vi "Scan for incomplete relaxations and re-submit script.vi"() -> ()   [LabVIEW 2010]
panel:
  in  "Move to other folder in source":bool
  in  "Target Directory":path=path "D:/Ab-initio/VASP Calcs/2D_Grain Boundaries/Batch25_20130914"
  in  "Source Directory":path=path "D:/Ab-initio/VASP Calcs/2D_Grain Boundaries/Batch18_20130828/A3B12_Periodic_Twin/CONTCAR"
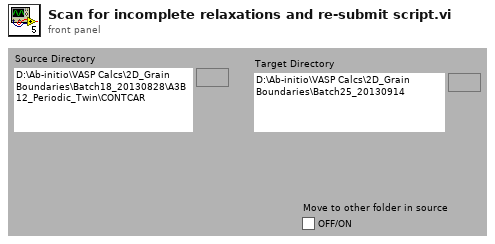
[diagram p1: front panel]
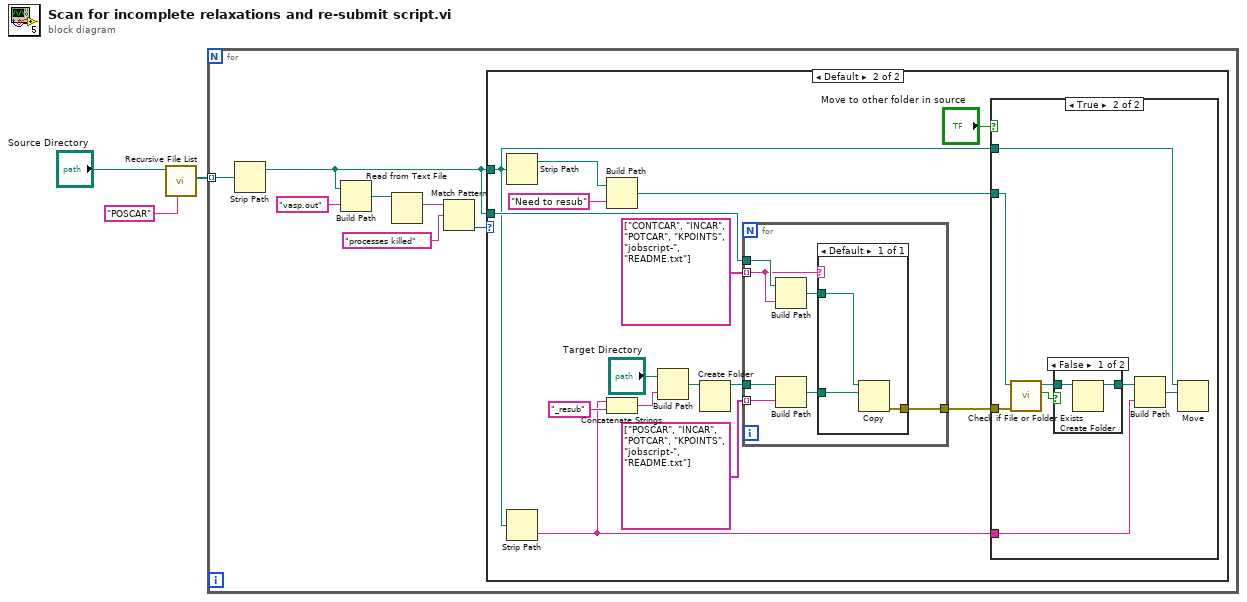
[diagram p0: block diagram]
diagram:
  n1 = call <vilib>:"Recursive File List.vi"("pattern"="POSCAR", "Folder Path"="Source Directory") -> ("All Files in Dir"=w1:path[])  [unwired: 5 in, 4 out]
  n2 = for {
    tunnel: w1 -> [w10] mode=indexing
    n3 = Strip Path(path=w10) -> (stripped path=w4:path)  [unwired: 1 out]
    n4 = Build Path(base path=w4, name or relative path="vasp.out") -> (appended path=w8:path)
    n5 = Read from Text File(file (use dialog)=w8) -> (text=w7:string)  [unwired: 3 in, 3 out]
    n6 = Match Pattern(string=w7, regular expression="processes killed") -> (offset past match=w5:i32)  [unwired: 1 in, 3 out]
    n7 = case shown="Default" w5 {
      tunnel: w4 -> [_ w21]
      tunnel: w4 -> [_ w14]
      frame -1 {
      }
      frame Default {
        n8 = Strip Path(path=w14) -> (stripped path=w13:path)  [unwired: 1 out]
        n9 = Strip Path(path=w14) -> (name=w12:string)  [unwired: 1 out]
        n10 = Build Path(base path=w13, name or relative path="Need to resub") -> (appended path=w16:path)
        n11 = Concatenate Strings(w12, "_resub" ("string")) -> (w25:string)
        n12 = Build Path(base path="Target Directory", name or relative path=w25) -> (appended path=w19:path)
        n13 = Create Folder(path (use dialog)=w19) -> (created path=w22:path)  [unwired: 2 in, 2 out]
        n14 = for {
          tunnel: w21 -> [w43]
          tunnel: w22 -> [w41]
          tunnel: string[] ["CONTCAR", "INCAR", "POTCAR", "KPOINTS", "jobscript-", "README.txt"] -> [w38] mode=indexing
          tunnel: string[] ["POSCAR", "INCAR", "POTCAR", "KPOINTS", "jobscript-", "README.txt"] -> [w39] mode=indexing
          tunnel: [w37] -> w11
          n15 = Build Path(base path=w43, name or relative path=w38) -> (appended path=w42:path)
          n16 = Build Path(base path=w41, name or relative path=w39) -> (appended path=w40:path)
          n17 = case shown="Default" w38 {
            tunnel: w42 -> [w46]
            tunnel: w40 -> [w45]
            tunnel: [w44] -> w37
            frame Default {
              n18 = Copy(10:w45, 11:w46) -> (0:w44:errorcluster)  [unwired: 3 in, 2 out]
            }
          }
        }
        n19 = case shown="True" "Move to other folder in source" {
          tunnel: w16 -> [_ w29]
          tunnel: w14 -> [_ w33]
          tunnel: w12 -> [_ w31]
          tunnel: w11 -> [_ w26]
          frame False {
          }
          frame True {
            n20 = call <vilib>:"Check if File or Folder Exists.vi"("error in (no error)"=w26, "path"=w29) -> ("file or folder exists?"=w27:bool, "dup path"=w28:path)  [unwired: 7 in, 1 out]
            n21 = case shown="False" w27 {
              tunnel: [w35 w36] -> w32
              tunnel: w28 -> [w34 w36]
              frame False {
                n22 = Create Folder(path (use dialog)=w34) -> (created path=w35:path)  [unwired: 2 in, 2 out]
              }
              frame True {
              }
            }
            n23 = Build Path(base path=w32, name or relative path=w31) -> (appended path=w30:path)
            n24 = Move(source path=w33, 10:w30) -> ()  [unwired: 3 in, 3 out]
          }
        }
      }
    }
  }
